vi "Create Lossless Endpoint.vi"(7 "Refs":T1, 8 "error in (no error)":errorcluster, 10 "Type Descriptor":T2, 11 "Channel Term":refnum<vi>) -> (0 "error out":errorcluster, 3 "Element Term":refnum<vi>)   [LabVIEW 2022 SP3, in "FlexBlocks Support.lvlib"]
uses:
  FlexBlocks Support.lvlib
  Type Descriptor.ctl
  Terminal Direction.ctl
  Value Mode.ctl
  Special Terminal.ctl
  SM Refs.ctl
  <vilib>/Utility/miscctls.llb/LVPointTypeDef.ctl
  Status Terminals.ctl
  Lossless Terminals.ctl
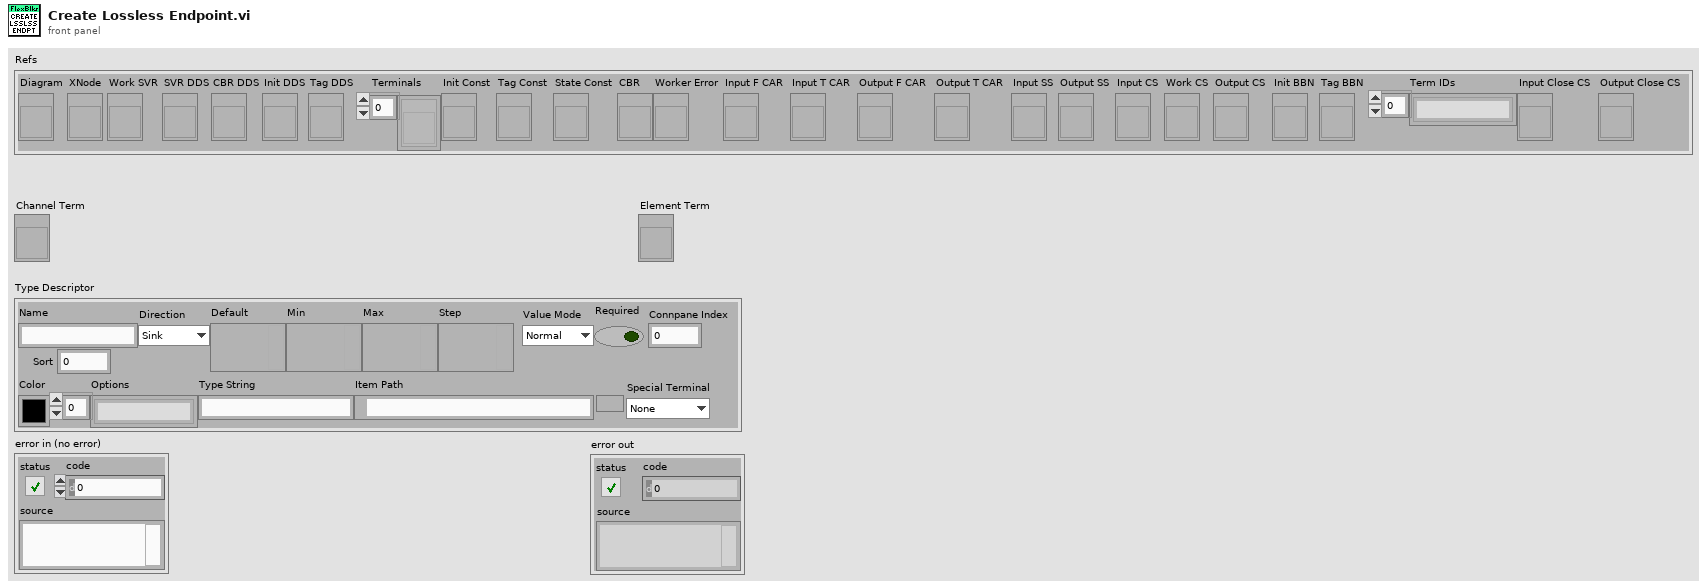
[diagram p1: front panel]
types:
  T1 = typedef "FlexBlocks Support.lvlib/SM Refs.ctl" = cluster{"Diagram":refnum<vi>, "XNode":refnum<vi>, "Work SVR":refnum<vi>, "SVR DDS":refnum<vi>, "CBR DDS":refnum<vi>, "Init DDS":refnum<vi>, "Tag DDS":refnum<vi>, "Terminals":refnum<vi>[], "Init Const":refnum<vi>, "Tag Const":refnum<vi>, "State Const":refnum<vi>, "CBR":refnum<vi>, "Worker Error":refnum<vi>, "Input F CAR":refnum<vi>, "Input T CAR":refnum<vi>, "Output F CAR":refnum<vi>, "Output T CAR":refnum<vi>, "Input SS":refnum<vi>, "Output SS":refnum<vi>, "Input CS":refnum<vi>, "Work CS":refnum<vi>, "Output CS":refnum<vi>, "Init BBN":refnum<vi>, "Tag BBN":refnum<vi>, "Term IDs":string[], "Input Close CS":refnum<vi>, "Output Close CS":refnum<vi>}
  T2 = typedef "FlexBlocks Support.lvlib/Type Descriptor.ctl" = cluster{"Name":string, "Direction":T3, "Default":variant, "Min":variant, "Max":variant, "Step":variant, "Value Mode":T4, "Color":u32, "Options":string[], "Type String":string, "Item Path":path, "Required":bool, "Connpane Index":i32, "Special Terminal":T5, "Sort":i32}
  T3 = typedef "FlexBlocks Support.lvlib/Terminal Direction.ctl" = enum16{"Sink", "Source"}
  T4 = typedef "FlexBlocks Support.lvlib/Value Mode.ctl" = enum16{"Normal", "Range", "Select"}
  T5 = typedef "FlexBlocks Support.lvlib/Special Terminal.ctl" = enum16{"None", "Action", "Init", "Tag", "State in", "State out", "Error"}
  T6 = typedef "FlexBlocks Support.lvlib/Lossless Terminals.ctl" = enum16{"Depth", "Timeout mS", "FlexChannel", "Release", "Restart", "Paused?", "Timed Out?", "Element", "Close", "Closed?"}
  T7 = typedef "FlexBlocks Support.lvlib/Status Terminals.ctl" = enum16{"# Pending Write", "# Pending Read", "Usage Ratio", "Queued Count", "Closed?", "Updated", "NC 6", "Sequence", "NC 8", "NC 9", "NC 10", "FlexChannel"}
  T8 = typedef "LVPointTypeDef.ctl" = cluster{"Horizontal":i16, "Vertical":i16}
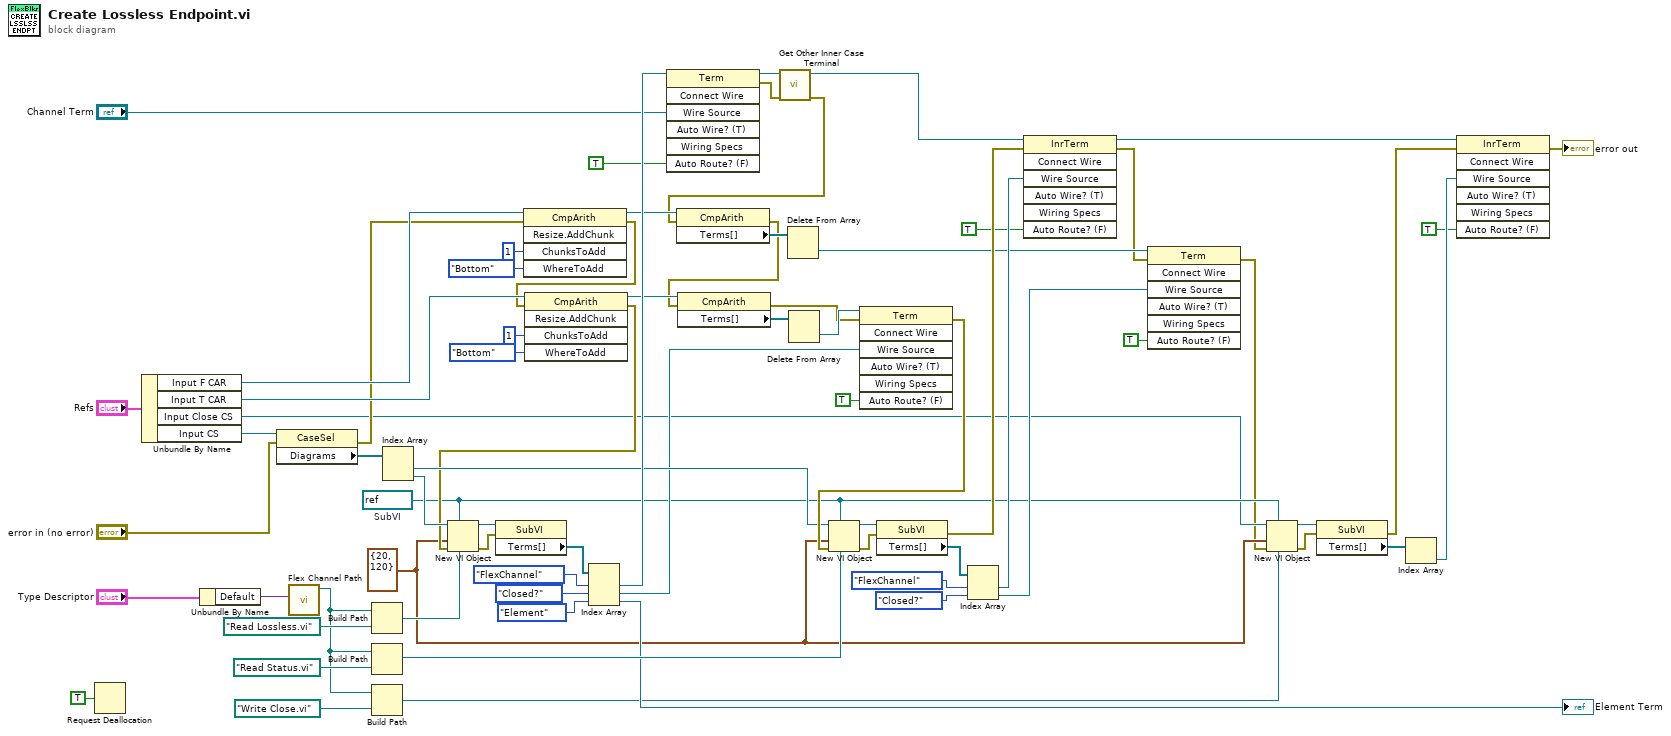
[diagram p0: block diagram]
diagram:
  w8 = T8 {"Horizontal"=20, "Vertical"=120} ("location")
  w9 = refnum<vi> refnum  # SubVI
  n1 = Request Deallocation(TRUE ("flag")) -> ()
  n2 = Unbundle By Name("Refs") -> ("Input F CAR"=w35:refnum<vi>, "Input T CAR"=w46:refnum<vi>, "Input Close CS"=w3:refnum<vi>, "Input CS"=w59:refnum<vi>)
  n3 = Unbundle By Name("Type Descriptor") -> ("Default"=w70:variant)
  n4 = property class="CaseSel"(reference=w59, error in="error in (no error)") -> (error out=w23:errorcluster, "Diagrams"=w58:refnum<vi>[])  [unwired: 1 out]
  n5 = call "Flex Channel Path.vi"("Variant"=w70) -> ("Channel Folder Path"=w5:path)  [unwired: 9 in, 1 out]
  n6 = Build Path(base path=w5, name or relative path=path "Read Lossless.vi") -> (appended path=w66:path)
  n7 = Build Path(base path=w5, name or relative path=path "Read Status.vi") -> (appended path=w54:path)
  n8 = Build Path(base path=w5, name or relative path=path "Write Close.vi") -> (appended path=w4:path)
  n9 = Index Array(array=w58) -> (element #1=w43:refnum<vi>, element #2=w57:refnum<vi>)  [unwired: 2 in]
  n10 = invoke class="CmpArith" method="Resize.AddChunk"(reference=w35, error in=w23, "ChunksToAdd"=u8 1 ("Chunks To Add"), "WhereToAdd"=enum8{"Bottom", "Top"}."Bottom" ("Where To Add")) -> (reference out=w34:refnum<vi>, error out=w22:errorcluster)  [unwired: 1 in, 3 out]
  n11 = invoke class="CmpArith" method="Resize.AddChunk"(reference=w46, error in=w22, "ChunksToAdd"=u8 1 ("Chunks To Add"), "WhereToAdd"=enum8{"Bottom", "Top"}."Bottom" ("Where To Add")) -> (reference out=w42:refnum<vi>, error out=w21:errorcluster)  [unwired: 1 in, 3 out]
  n12 = New VI Object(vi object class=w9, owner refnum=w57, position/next to=w8, 6:w66, 8:w21) -> (object refnum=w65:refnum<vi>, 0:w64:errorcluster)  [unwired: 3 in]
  n13 = property class="SubVI"(reference=w65, error in=w64) -> ("Terms[]"=w63:refnum<vi>[])  [unwired: 2 out]
  n14 = Index Array(array=w63, index #1=Lossless_Terminals."FlexChannel" ("Lossless Terminals"), index #2=Lossless_Terminals."Closed?" ("Lossless Terminals"), index #3=Lossless_Terminals."Element" ("Lossless Terminals")) -> (element #1=w62:refnum<vi>, element #2=w17:refnum<vi>, element #3=→"Element Term":refnum<vi>)
  n15 = invoke class="Term" method="Connect Wire"(reference=w62, "Wire Source"="Channel Term", "Auto Route? (F)"=TRUE) -> (reference out=w52:refnum<vi>, error out=w51:errorcluster)  [unwired: 4 in, 5 out]
  n16 = call "Get Other Inner Case Terminal.vi"("error in (no error)"=w51, "Term"=w52) -> ("error out"=w27:errorcluster, "Other InnerTerm"=w48:refnum<vi>)  [unwired: 8 in]
  n17 = property class="CmpArith"(reference=w34, error in=w27) -> (error out=w26:errorcluster, "Terms[]"=w38:refnum<vi>[])  [unwired: 1 out]
  n18 = property class="CmpArith"(reference=w42, error in=w26) -> (error out=w25:errorcluster, "Terms[]"=w41:refnum<vi>[])  [unwired: 1 out]
  n19 = Delete From Array(array=w38) -> (deleted portion=w31:refnum<vi>)  [unwired: 2 in, 1 out]
  n20 = Delete From Array(array=w41) -> (deleted portion=w40:refnum<vi>)  [unwired: 2 in, 1 out]
  n21 = invoke class="Term" method="Connect Wire"(reference=w40, error in=w25, "Wire Source"=w17, "Auto Route? (F)"=TRUE) -> (error out=w73:errorcluster)  [unwired: 3 in, 6 out]
  n22 = New VI Object(vi object class=w9, owner refnum=w43, position/next to=w8, 6:w54, 8:w73) -> (object refnum=w55:refnum<vi>, 0:w56:errorcluster)  [unwired: 3 in]
  n23 = property class="SubVI"(reference=w55, error in=w56) -> (error out=w33:errorcluster, "Terms[]"=w53:refnum<vi>[])  [unwired: 1 out]
  n24 = Index Array(array=w53, index #1=Status_Terminals."FlexChannel" ("Status Terminals"), index #2=Status_Terminals."Closed?" ("Status Terminals")) -> (element #1=w47:refnum<vi>, element #2=w28:refnum<vi>)
  n25 = invoke class="InrTerm" method="Connect Wire"(reference=w48, error in=w33, "Wire Source"=w47, "Auto Route? (F)"=TRUE) -> (reference out=w1:refnum<vi>, error out=w30:errorcluster)  [unwired: 3 in, 5 out]
  n26 = invoke class="Term" method="Connect Wire"(reference=w31, error in=w30, "Wire Source"=w28, "Auto Route? (F)"=TRUE) -> (error out=w2:errorcluster)  [unwired: 3 in, 6 out]
  n27 = New VI Object(vi object class=w9, owner refnum=w3, position/next to=w8, 6:w4, 8:w2) -> (object refnum=w15:refnum<vi>, 0:w14:errorcluster)  [unwired: 3 in]
  n28 = property class="SubVI"(reference=w15, error in=w14) -> (error out=w11:errorcluster, "Terms[]"=w13:refnum<vi>[])  [unwired: 1 out]
  n29 = Index Array(array=w13) -> (element=w12:refnum<vi>)  [unwired: 1 in]
  n30 = invoke class="InrTerm" method="Connect Wire"(reference=w1, error in=w11, "Wire Source"=w12, "Auto Route? (F)"=TRUE) -> (error out=→"error out":errorcluster)  [unwired: 3 in, 6 out]
